vi "ITECH_Example.vi"() -> ()   [LabVIEW 2015]
uses:
  <instrlib>/IT6000C/IT6000C.lvlib
panel:
  in  "Serial Configuration":T1={"Baud Rate"=9600, "Parity"=0, "Data Bits"=8, "Stop Bits"=10, "Flow Control"=0} {"Flow Control" items=["None", "XON/XOFF", "RTS/CTS", "XON/XOFF & RTS/CTS", "DTR/DSR", "XON/XOFF & DTR/DSR"]; "Stop Bits" items=["1.0"=10, "1.5"=15, "2.0"=20]; "Data Bits" items=["7"=7, "8"=8]; "Parity" items=["None", "Odd", "Even", "Mark", "Space"]; "Baud Rate" items=["300"=300, "600"=600, "1200"=1200, "2400"=2400, "4800"=4800, "9600"=9600, "19200"=19200]}
  out "电流回读值(A)":dbl format="%.2g"
  out "电压回读值(V)":dbl format="%.2g"
  in  "输出打开or关闭":bool=TRUE
  in  "电流设定值":dbl
  in  "电压设定值":dbl
  in  "error in (no error)":errorcluster
  in  "VISA resource name":refnum<visa-resource-name>
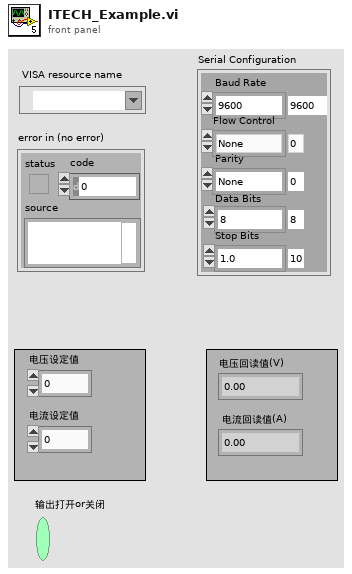
[diagram p1: front panel]
types:
  T1 = cluster{"Baud Rate":u32, "Parity":u16, "Data Bits":u16, "Stop Bits":u16, "Flow Control":u16}
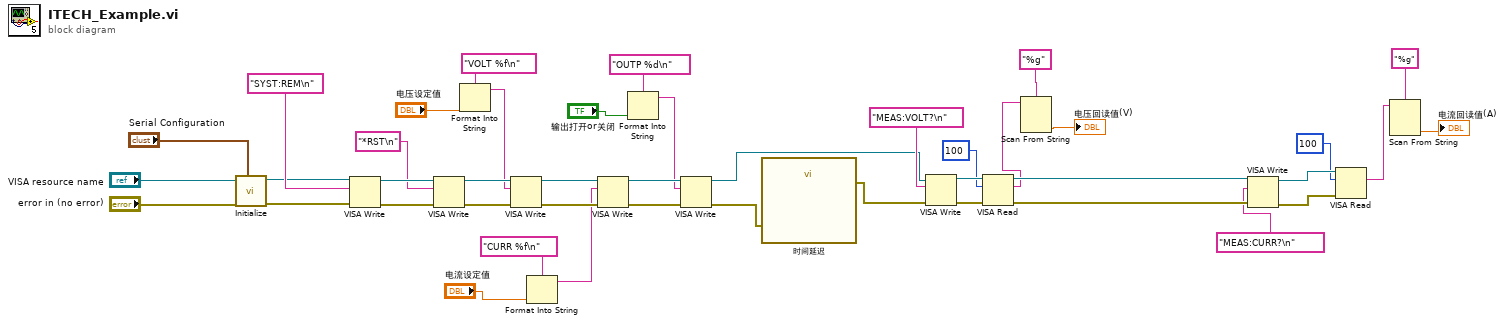
[diagram p0: block diagram]
diagram:
  n1 = call <instrlib>:"Initialize.vi"("Serial Configuration"="Serial Configuration", "error in (no error)"="error in (no error)", "VISA resource name"="VISA resource name") -> ("error out"=w2:errorcluster, "VISA resource name out"=w3:refnum<visa-resource-name>)  [unwired: 7 in]
  n2 = VISA Write(VISA resource name=w3, write buffer="SYST:REM\n", error in (no error)=w2) -> (VISA resource name out=w41:refnum<visa-resource-name>, error out=w42:errorcluster)  [unwired: 1 out]
  n3 = VISA Write(VISA resource name=w41, write buffer="*RST\n", error in (no error)=w42) -> (VISA resource name out=w39:refnum<visa-resource-name>, error out=w38:errorcluster)  [unwired: 1 out]
  n4 = Format Into String(format string="VOLT %f\n" ("Command"), "电压设定值") -> (resulting string=w26:string)  [unwired: 2 in, 1 out]
  n5 = VISA Write(VISA resource name=w39, write buffer=w26, error in (no error)=w38) -> (VISA resource name out=w33:refnum<visa-resource-name>, error out=w32:errorcluster)  [unwired: 1 out]
  n6 = Format Into String(format string="CURR %f\n" ("Command"), "电流设定值") -> (resulting string=w25:string)  [unwired: 2 in, 1 out]
  n7 = VISA Write(VISA resource name=w33, write buffer=w25, error in (no error)=w32) -> (VISA resource name out=w30:refnum<visa-resource-name>, error out=w29:errorcluster)  [unwired: 1 out]
  n8 = Format Into String(format string="OUTP %d\n" ("Command"), "输出打开or关闭") -> (resulting string=w27:string)  [unwired: 2 in, 1 out]
  n9 = VISA Write(VISA resource name=w30, write buffer=w27, error in (no error)=w29) -> (VISA resource name out=w7:refnum<visa-resource-name>, error out=w9:errorcluster)  [unwired: 1 out]
  n10 = call "时间延迟"("error in (no error)"=w9) -> ("error out"=w8:errorcluster)  [unwired: 10 in]
  n11 = VISA Write(VISA resource name=w7, write buffer="MEAS:VOLT?\n" ("Voltage Measurement Command"), error in (no error)=w8) -> (VISA resource name out=w23:refnum<visa-resource-name>, error out=w24:errorcluster)  [unwired: 1 out]
  n12 = VISA Read(VISA resource name=w23, byte count=u32 100, error in (no error)=w24) -> (VISA resource name out=w18:refnum<visa-resource-name>, read buffer=w10:string, error out=w17:errorcluster)  [unwired: 1 out]
  n13 = Scan From String(format string="%g", input string=w10) -> (output 1=→"电压回读值(V)":dbl)  [unwired: 3 in, 3 out]
  n14 = VISA Write(VISA resource name=w18, write buffer="MEAS:CURR?\n" ("Current Measurement Command"), error in (no error)=w17) -> (VISA resource name out=w16:refnum<visa-resource-name>, error out=w15:errorcluster)  [unwired: 1 out]
  n15 = VISA Read(VISA resource name=w16, byte count=u32 100, error in (no error)=w15) -> (read buffer=w11:string)  [unwired: 3 out]
  n16 = Scan From String(format string="%g", input string=w11) -> (output 1=→"电流回读值(A)":dbl)  [unwired: 3 in, 3 out]
